vi "PLC_Receive.vi"(8 "error in (no error)":errorcluster, 11 "VISA resource name":refnum<visa-resource-name>="COM13") -> (0 "error out":errorcluster, 1 "loops(29)":i32, 2 "fail?":bool, 3 "pass?":bool)   [LabVIEW 2011]
uses:
  <vilib>/Instr/_visa.llb/VISA Configure Serial Port (Instr).vi
panel:
  out "String":string
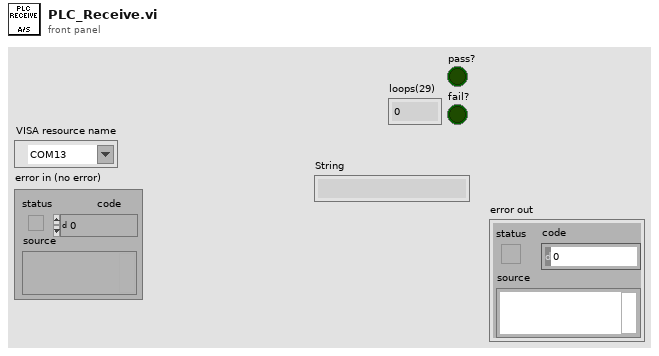
[diagram p1: front panel]
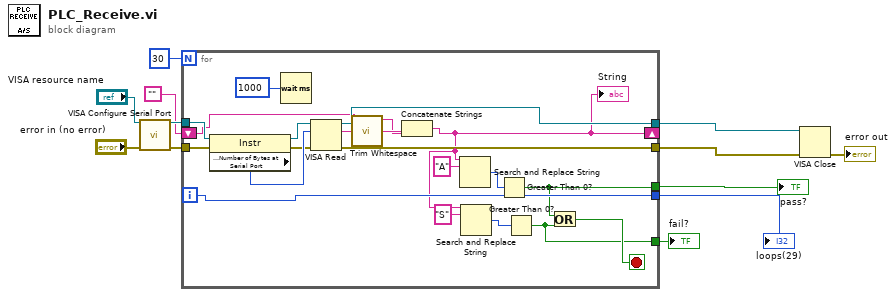
[diagram p0: block diagram]
diagram:
  n1 = call-poly "VISA Configure Serial Port"("VISA resource name"="VISA resource name", "error in (no error)"="error in (no error)") -> ("VISA resource name out"=w11:refnum<visa-resource-name>, "error out"=w10:errorcluster)  [unwired: 12 in]
  n2 = for {
    N: 30 -> [_]
    tunnel: w11 -> [w32]
    tunnel: w10 -> [w31]
    tunnel: [w27] -> w9
    tunnel: [w26] -> w8
    tunnel: [w23] -> w4
    shift-right: [w13] -> _
    shift-left: "" -> [w21]
    tunnel: [w15] -> w2
    tunnel: [w14] -> w1
    i -> [w23]
    stop <- w16 stop-if-true
    n3 = property class="Instr"(reference=w32, error in=w31) -> (reference out=w30:refnum<visa-resource-name>, error out=w28:errorcluster, "Serial Settings:Number of Bytes at Serial Port"=w29:u32)
    n4 = Wait (ms)(milliseconds to wait=u32 1000) -> ()  [unwired: 1 out]
    n5 = VISA Read(VISA resource name=w30, byte count=w29, error in (no error)=w28) -> (VISA resource name out=w27:refnum<visa-resource-name>, read buffer=w24:string, error out=w26:errorcluster)  [unwired: 1 out]
    n6 = call <vilib>:"Trim Whitespace.vi"("string"=w24) -> ("trimmed string"=w22:string)  [unwired: 1 in]
    n7 = Concatenate Strings(w22, w21) -> (w13:string)
    "String" <- w13
    n8 = Search and Replace String(input string=w13, search string="A") -> (number of replacements=w19:i32)  [unwired: 6 in, 3 out]
    n9 = Search and Replace String(input string=w13, search string="S") -> (number of replacements=w17:i32)  [unwired: 6 in, 3 out]
    n10 = Greater Than 0?(x=w19) -> (x > 0?=w15:bool)
    n11 = Greater Than 0?(x=w17) -> (x > 0?=w14:bool)
    n12 = Or(x=w15, y=w14) -> (x .or. y?=w16:bool)
  }
  "loops(29)" <- w4
  "pass?" <- w2
  "fail?" <- w1
  n13 = VISA Close(VISA resource name=w9, error in (no error)=w8) -> (error out=→"error out":errorcluster)
